vi "Write Error.vi"(8 "error in (no error)":errorcluster, 10 "Error":bool, 11 "MySQL initial erroe in":refnum<class "MySQL initial error.lvclass">) -> (0 "error out":errorcluster, 3 "MySQL initial erroe out":refnum<class "MySQL initial error.lvclass">)   [LabVIEW 2019, in "DataBase.lvlib" / "MySQL initial error.lvclass"]
uses:
  MySQL initial error.lvclass
  MySQL initial error.lvclass/MySQL initial error.ctl
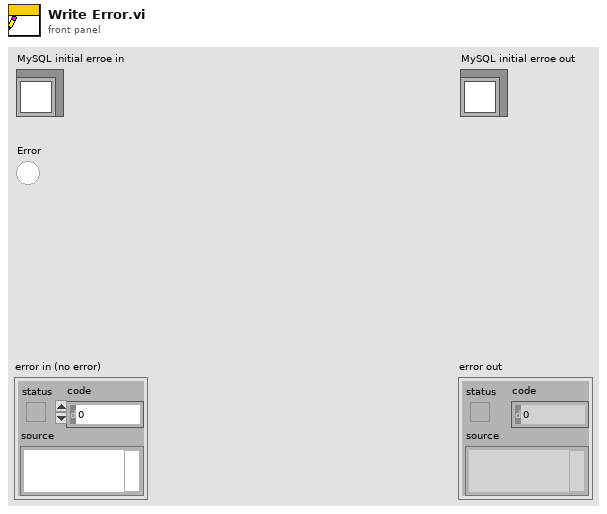
[diagram p1: front panel]
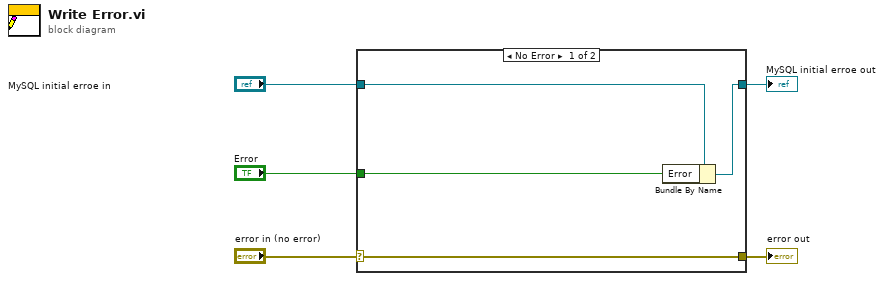
[diagram p0: block diagram]
diagram:
  n1 = case shown="No Error" "error in (no error)" {
    selector: "error in (no error)" -> [w9 w10]
    tunnel: [w9 w10] -> w4
    tunnel: [w7 w11] -> w2
    tunnel: "MySQL initial erroe in" -> [w8 w11]
    tunnel: "Error" -> [w6 _]
    frame No Error {
      n2 = Bundle By Name(cluster=w8, "Error"=w6) -> (w7:refnum<class "MySQL initial error.lvclass">)
    }
    frame Error {
    }
  }
  "error out" <- w4
  "MySQL initial erroe out" <- w2
